vi "VM_ProjetoV4.vi"() -> ()   [LabVIEW 2016]
uses:
  <vilib>/vision/driver/NI_Vision_Acquisition_Software.lvlib
  <resource>/objmgr/imaqdx.rc
  <vilib>/Analysis/NI_AALBase.lvlib
  <vilib>/Analysis/baseanly.llb/Mean (DBL).vi
  <vilib>/userdefined/High Color/IMAQdx.ctl
panel:
  out "Bayer Parameters":T1={"Pattern"=0, "Algorithm"=0, "Red Gain"=1.0, "Green Gain"=1.0, "Blue Gain"=1.0} {"Blue Gain" format="%_4g"; "Green Gain" format="%_4g"; "Red Gain" format="%_4g"; "Algorithm" items=["Bilinear", "VNG"]; "Pattern" items=["GB", "GR", "BG", "RG"]}
  out "output cluster":T2
  in  "Cut Limit":dbl=55.0 format="%#_13g"
  in  "Confirma":bool
  out "Status":string
  out "Câmera Robo":T3(plugin-control)
  out "Câmera Mesa":T3(plugin-control)
  in  "Começa jogada":bool
  in  "stop":bool
  in  "Source Câmera Robo":T4
  in  "Source Câmera Mesa":T4
  out "Dobrao":bool
  out "Passa Vez":bool
  out "place pos Norm":dbl[](array[numeric])
  out "pick pos Norm":dbl[](array[numeric])
  out "place angle":dbl
  out "pick angle":dbl
  # "x 91\ny 176"
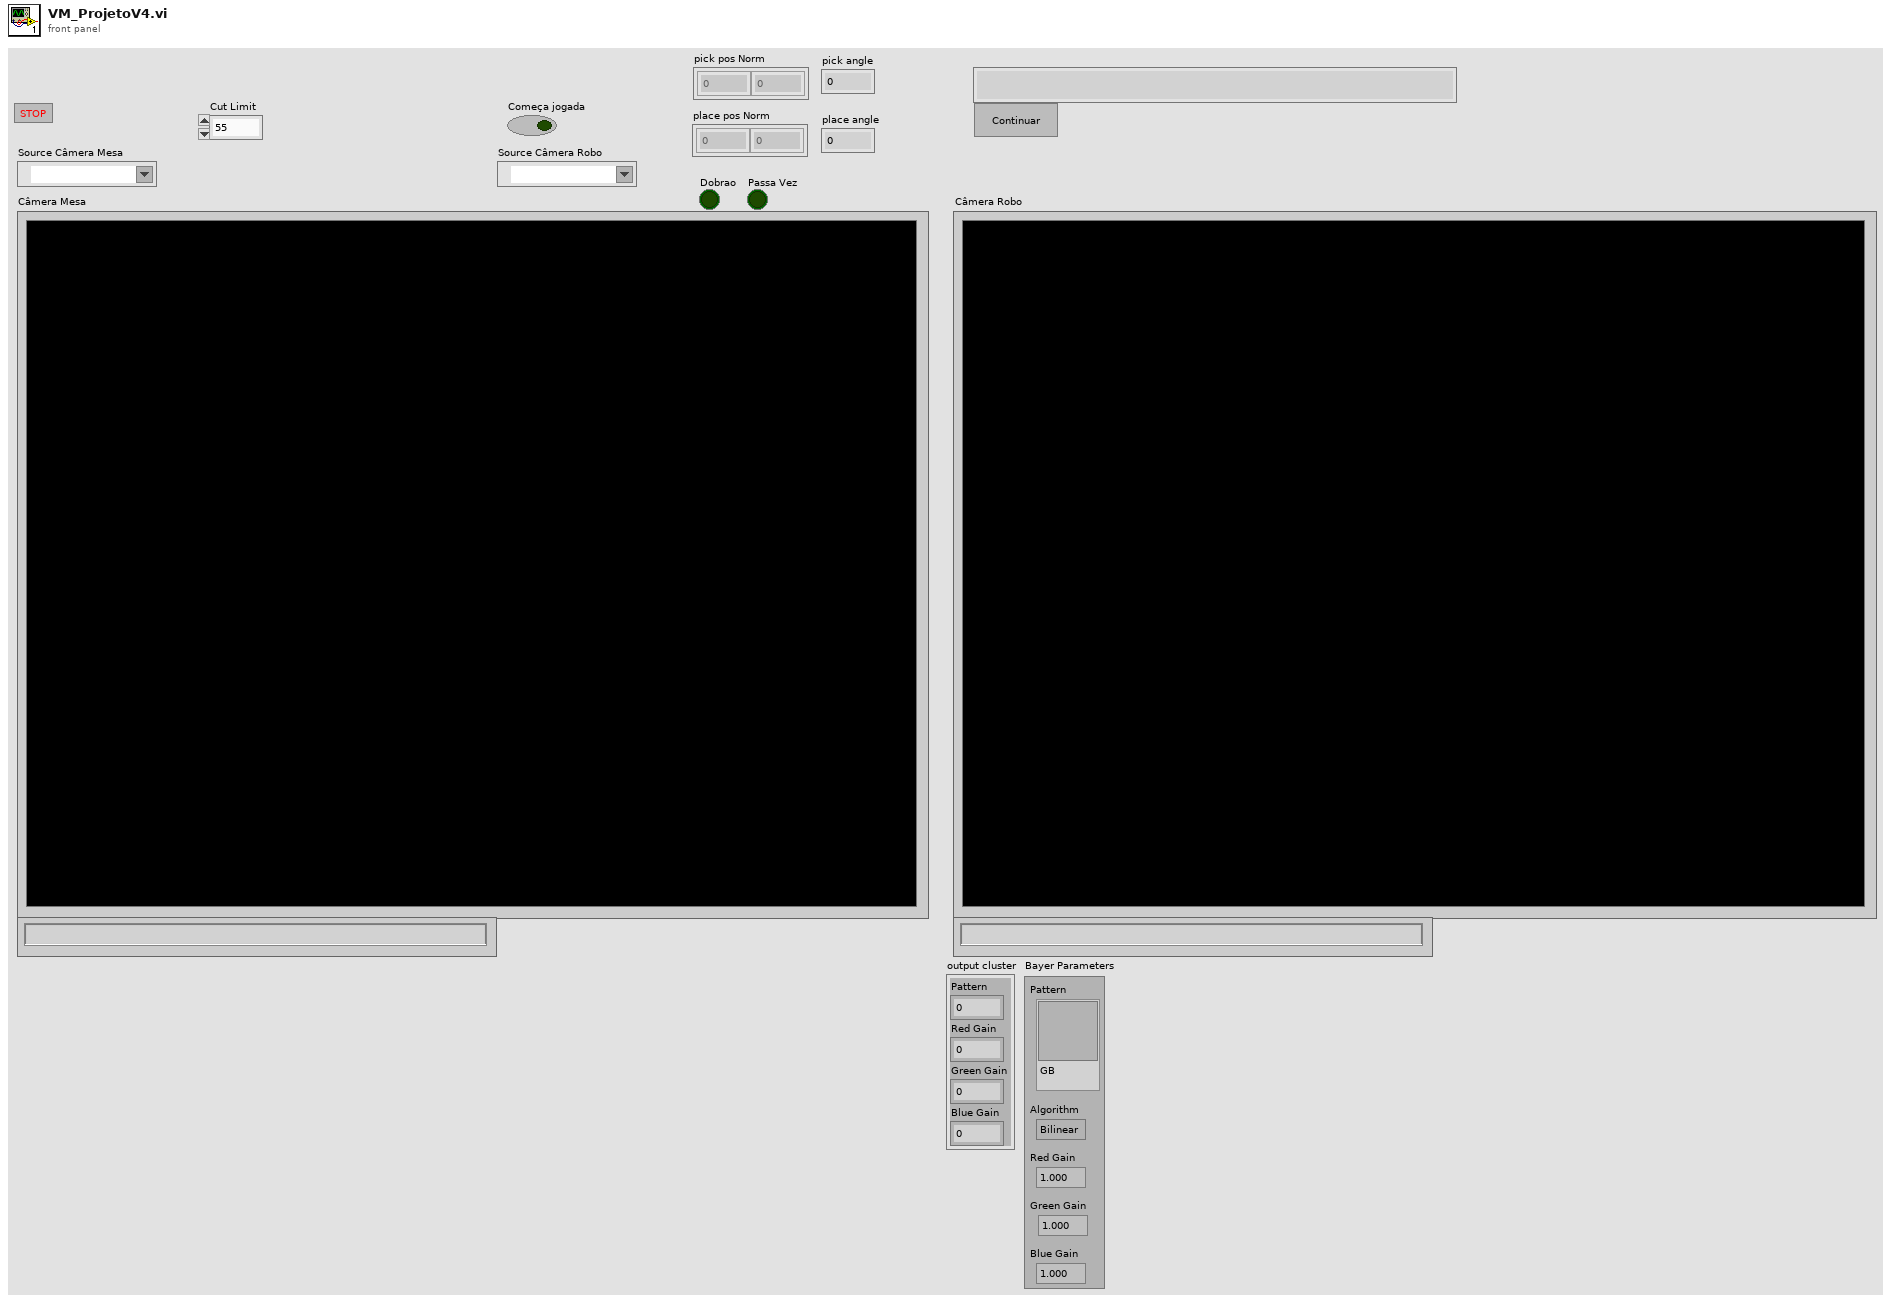
[diagram p1: front panel]
types:
  T1 = cluster{"Pattern":i32, "Algorithm":i32, "Red Gain":dbl, "Green Gain":dbl, "Blue Gain":dbl}
  T2 = cluster{"Pattern":i32, "Red Gain":fxp<+,16,2>, "Green Gain":fxp<+,16,2>, "Blue Gain":fxp<+,16,2>}
  T3 = typedef "IMAQ Image.ctl" = refnum<image>
  T4 = typedef "IMAQdx.ctl" = refnum<k21>
  T5 = typedef "IMAQ Rectangle" = cluster{"Left":i32, "Top":i32, "Right":i32, "Bottom":i32, "Rotation":dbl}
  T6 = typedef "ROI Descriptor" = cluster{"Global Rectangle":i32[], "Contours":cluster{"ID":enum32{"External", "Internal"}, "Type":u32, "Coordinates":i32[]}[]}
  T7 = cluster{"Position":cluster{"x":sgl, "y":sgl}, "Angle":sgl, "Scale":sgl, "Score":sgl, "Bounding Box":cluster{"x":sgl, "y":sgl}[]}[]
  T8 = cluster{"Centro Peça":dbl[], "Centros Númeors":dbl[][], "Números":u8[], "ROI Números":T6[]}[]
  T9 = cluster{"Centro Peça":dbl[], "Centros Númeors":dbl[][], "Números":u8[], "ROI Números":T6[]}
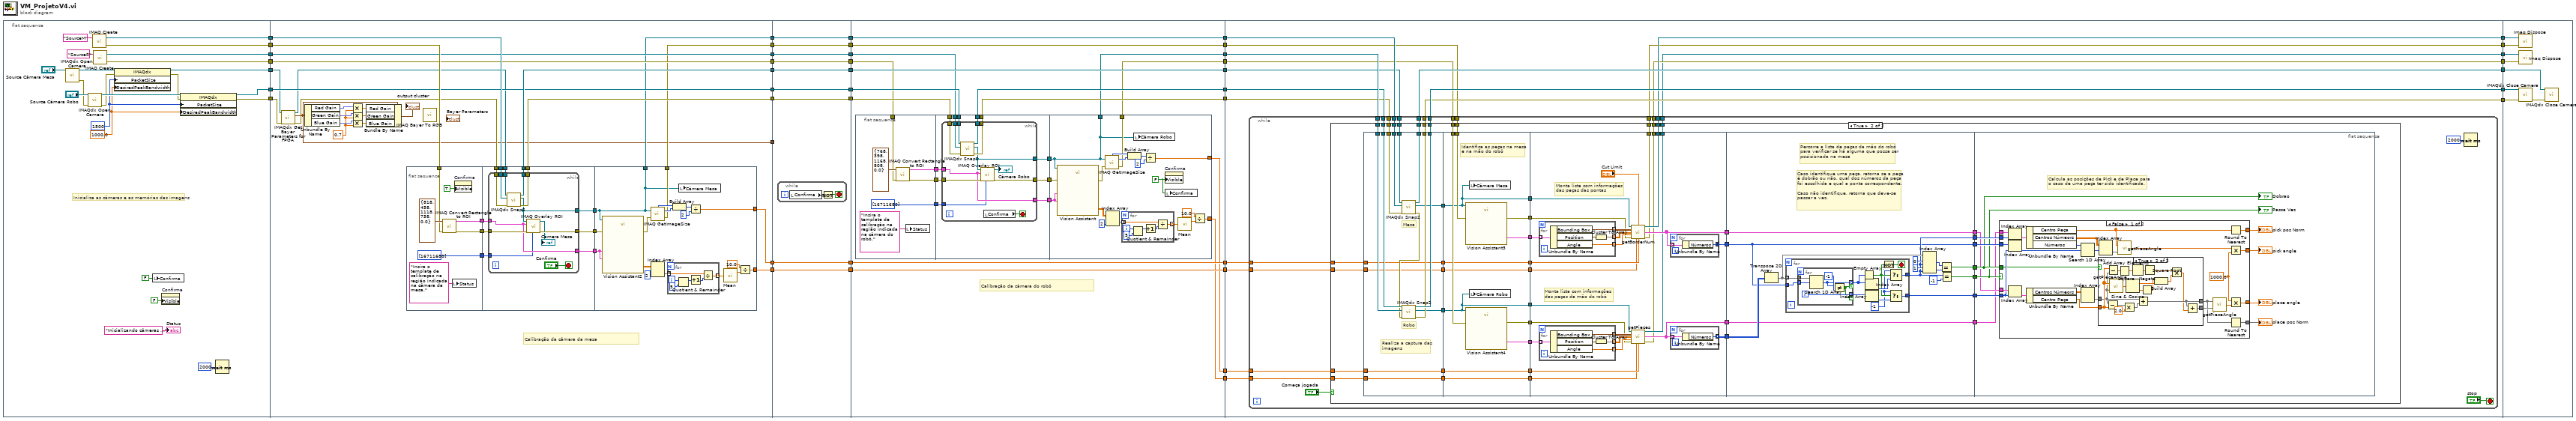
[diagram p0: block diagram]
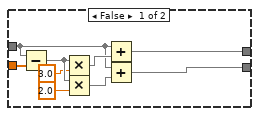
[diagram p3: hidden frame]
diagram:
  n1 = flat-sequence {
    tunnel: [w62] -> w37
    tunnel: [w61] -> w36
    tunnel: [w56] -> w35
    tunnel: [w60] -> w34
    tunnel: [w59] -> w33
    tunnel: [w55] -> w32
    tunnel: [w46] -> w31
    tunnel: w37 -> [w93]
    tunnel: w36 -> [w94]
    tunnel: w35 -> [w79]
    tunnel: w34 -> [w90]
    tunnel: w33 -> [w89]
    tunnel: w32 -> [w77]
    tunnel: [w84] -> w19
    tunnel: [w83] -> w17
    tunnel: [w90] -> w15
    tunnel: [w89] -> w13
    tunnel: [w88] -> w11
    tunnel: [w87] -> w9
    tunnel: w31 -> [w87]
    tunnel: [w86] -> w7
    tunnel: [w81] -> w5
    tunnel: [w80] -> w3
    tunnel: [w68] -> w1
    tunnel: w19 -> [w158]
    tunnel: [w158] -> w18
    tunnel: w17 -> [w157]
    tunnel: [w157] -> w16
    tunnel: w15 -> [w156]
    tunnel: [w156] -> w14
    tunnel: w13 -> [w155]
    tunnel: [w155] -> w12
    tunnel: w11 -> [w154]
    tunnel: [w154] -> w10
    tunnel: w9 -> [w153]
    tunnel: [w153] -> w8
    tunnel: w7 -> [w152]
    tunnel: [w152] -> w6
    tunnel: w5 -> [w151]
    tunnel: [w151] -> w4
    tunnel: w3 -> [w150]
    tunnel: [w150] -> w2
    tunnel: w1 -> [_]
    tunnel: w18 -> [w181]
    tunnel: [w181] -> w30
    tunnel: w16 -> [w180]
    tunnel: [w180] -> w29
    tunnel: w14 -> [w166]
    tunnel: [w165] -> w28
    tunnel: w12 -> [w164]
    tunnel: [w163] -> w27
    tunnel: w10 -> [w179]
    tunnel: [w179] -> w26
    tunnel: w8 -> [w168]
    tunnel: [w167] -> w25
    tunnel: w6 -> [w170]
    tunnel: [w169] -> w24
    tunnel: w4 -> [w178]
    tunnel: [w178] -> w23
    tunnel: w2 -> [w177]
    tunnel: [w177] -> w22
    tunnel: [w162] -> w21
    tunnel: [w161] -> w20
    tunnel: [w249] -> w44
    tunnel: [w252] -> w43
    tunnel: [w246] -> w42
    tunnel: [w251] -> w41
    tunnel: [w250] -> w40
    tunnel: [w248] -> w39
    tunnel: [w247] -> w38
    tunnel: w30 -> [w245]
    tunnel: w29 -> [w244]
    tunnel: w28 -> [w243]
    tunnel: w27 -> [w242]
    tunnel: w26 -> [w241]
    tunnel: w25 -> [w240]
    tunnel: w24 -> [w239]
    tunnel: w23 -> [w237]
    tunnel: w22 -> [w238]
    tunnel: w21 -> [w235]
    tunnel: w20 -> [w236]
    tunnel: w44 -> [w488]
    tunnel: w43 -> [w486]
    tunnel: w42 -> [w490]
    tunnel: w41 -> [w493]
    tunnel: w40 -> [w492]
    tunnel: w39 -> [w489]
    tunnel: w38 -> [w491]
    frame #0 {
      w50 = 1000.0 ("DesiredPeakBandwidth")
      w51 = u32 1500 ("PacketSize")
      # "Inicializa as câmeras e as memórias das imagens"
      n2 = call <vilib>:"IMAQdx Open Camera.vi"("Session In"="Source Câmera Mesa") -> ("error out"=w54:errorcluster, "Session Out"=w57:T4)  [unwired: 9 in]
      n3 = call <vilib>:"IMAQdx Open Camera.vi"("error in"=w54, "Session In"="Source Câmera Robo") -> ("error out"=w53:errorcluster, "Session Out"=w58:T4)  [unwired: 8 in]
      n4 = call "IMAQ Create"("Image Name"="SourceM") -> ("New Image"=w62:T3, "error out"=w61:errorcluster)  [unwired: 4 in]
      n5 = call "IMAQ Create"("Image Name"="SourceR") -> ("New Image"=w60:T3, "error out"=w59:errorcluster)  [unwired: 4 in]
      n6 = property class="IMAQdx"(reference=w57, error in=w53, "PacketSize"=w51, "DesiredPeakBandwidth"=w50) -> (reference out=w56:T4, error out=w52:errorcluster)
      n7 = local write "Confirma"(FALSE ("Confirma")) -> ()
      n8 = property on="Confirma" class="Bool (strict)"("Visible"=FALSE) -> ()  [unwired: 2 in, 2 out]
      n9 = property class="IMAQdx"(reference=w58, error in=w52, "PacketSize"=w51, "DesiredPeakBandwidth"=w50) -> (reference out=w46:T4, error out=w55:errorcluster)
      n10 = Wait (ms)(milliseconds to wait=u32 2000) -> ()  [unwired: 1 out]
      "Status" <- "Inicializando câmeras ..." ("Status")
    }
    frame #1 {
      w69 = 0.7
      # "Calibração da câmera da mesa"
      n11 = call <vilib>:"IMAQdx Get Bayer Parameters for FPGA.vi"("error in (no error)"=w77, "IMAQdx Session In"=w79) -> ("error out"=w76:errorcluster, "Bayer Parameters"=w68:T2, "IMAQdx Session Out"=w78:T4)  [unwired: 7 in]
      n12 = Unbundle By Name(w68) -> ("Red Gain"=w72:fxp<+,16,2>, "Green Gain"=w71:fxp<+,16,2>, "Blue Gain"=w70:fxp<+,16,2>)
      n13 = Multiply(x=w72, y=w69) -> (x*y=w75:dbl)
      n14 = Multiply(x=w71, y=w69) -> (x*y=w74:dbl)
      n15 = Multiply(x=w70, y=w69) -> (x*y=w73:dbl)
      n16 = Bundle By Name(cluster=w68, "Red Gain"=w75, "Green Gain"=w74, "Blue Gain"=w73) -> (→"output cluster":T2)
      n17 = flat-sequence {
        tunnel: w94 -> [w101]
        tunnel: [w99] -> w96
        tunnel: [w98] -> w95
        tunnel: [u32[] [16711680] ("Colors (Green)")] -> w82
        tunnel: w78 -> [w114]
        tunnel: w76 -> [w113]
        tunnel: w93 -> [w112]
        tunnel: [w111] -> w88
        tunnel: [w110] -> w86
        tunnel: w96 -> [w109]
        tunnel: w95 -> [w108]
        tunnel: [w107] -> w92
        tunnel: [w106] -> w91
        tunnel: [w105] -> w85
        tunnel: w82 -> [w104]
        tunnel: w92 -> [w143]
        tunnel: w91 -> [w142]
        tunnel: [w134] -> w81
        tunnel: w85 -> [w127]
        tunnel: [w127] -> w84
        tunnel: [w129] -> w83
        tunnel: [w128] -> w80
        frame #0 {
          n18 = call "IMAQ Convert Rectangle to ROI"("error in (no error)"=w101, "Rectangle"=T5 {"Left"=818, "Top"=458, "Right"=1118, "Bottom"=758, "Rotation"=0.0}) -> ("error out"=w99:errorcluster, "ROI Descriptor"=w98:T6)  [unwired: 7 in]
          n19 = local write "Status"("Insira o template de calibração na região indicada na câmera da mesa." ("Status")) -> ()
          n20 = property on="Confirma" class="Bool (strict)"("Visible"=TRUE) -> ()  [unwired: 2 in, 2 out]
        }
        frame #1 {
          n21 = while {
            tunnel: w114 -> [w125]
            tunnel: w113 -> [w124]
            tunnel: w112 -> [w123]
            tunnel: [w122] -> w111
            tunnel: [w121] -> w110
            tunnel: w109 -> [w120]
            tunnel: w108 -> [w117]
            tunnel: [w119] -> w107
            tunnel: [w117] -> w106
            tunnel: [w116] -> w105
            tunnel: w104 -> [w115]
            stop <- "Confirma" stop-if-true
            n22 = call <vilib>:"IMAQdx Snap2.vi"("error in"=w124, "Image In"=w123, "Session In"=w125) -> ("error out"=w121:errorcluster, "Image Out"=w116:T3, "Session Out"=w122:T4)  [unwired: 6 in]
            n23 = call "IMAQ Overlay ROI"("Colors (Green)"=w115, "error in (no error)"=w120, "ROI Descriptor"=w117, "Image"=w116) -> ("error out"=w119:errorcluster, "Image Out"=→"Câmera Mesa":T3)  [unwired: 6 in]
          }
        }
        frame #2 {
          n24 = call "Vision Assistant2"("Image In"=w127, "ROI Descriptor (Adv. Straight Edge 1)"=w142, "ROI Descriptor (Copy of Adv. Straight Edge 1)"=w142, "error in"=w143) -> ("Caliper Results (Caliper 2)"=w141:sgl[][], "error out"=w135:errorcluster)  [unwired: 21 in, 1 out]
          n25 = call "IMAQ GetImageSize"("Image"=w127, "error in (no error)"=w135) -> ("Y Resolution"=w133:i32, "X Resolution"=w132:i32, "error out"=w129:errorcluster)  [unwired: 2 in]
          n26 = Index Array(array=w141, index (col)=2 ("disabled index (col)")) -> (element=w139:sgl[])  [unwired: 1 in]
          n27 = for {
            tunnel: w139 -> [w146] mode=indexing
            tunnel: [w144] -> w138 mode=indexing
            i -> [w149]
            n28 = Quotient & Remainder(x=w149, y=5) -> (x-y*floor(x/y)=w147:i32)  [unwired: 1 out]
            n29 = Increment(x=w147) -> (x+1=w145:i32)
            n30 = Divide(x=w146, y=w145) -> (x/y=w144:sgl)
          }
          n31 = Build Array(w132, w133) -> (w131:i32[])
          n32 = local write "Câmera Mesa"(w127) -> ()
          n33 = Divide(x=w131, y=2) -> (x/y=w128:dbl[])
          n34 = call-poly <vilib>:"Mean.vi"("X"=w138) -> ("mean"=w137:dbl)  [unwired: 1 out]
          n35 = Divide(x=10.0, y=w137) -> (x/y=w134:dbl)
        }
      }
      n36 = call "IMAQ Bayer To RGB"() -> ()  [unwired: 10 in, 2 out]
    }
    frame #2 {
      n37 = while {
        stop <- w160 stop-if-true
        n38 = local read "Confirma"() -> (w159:bool)
        n39 = Not(x=w159) -> (.not. x?=w160:bool)
      }
    }
    frame #3 {
      # "Calibração da câmera do robô"
      n40 = flat-sequence {
        tunnel: w164 -> [w185]
        tunnel: [w184] -> w176
        tunnel: [w183] -> w175
        tunnel: [u32[] [16711680] ("Colors (Green)")] -> w174
        tunnel: w168 -> [w198]
        tunnel: w170 -> [w197]
        tunnel: w166 -> [w196]
        tunnel: [w195] -> w167
        tunnel: [w194] -> w169
        tunnel: w176 -> [w193]
        tunnel: w175 -> [w192]
        tunnel: [w191] -> w173
        tunnel: [w190] -> w172
        tunnel: [w189] -> w171
        tunnel: w174 -> [w188]
        tunnel: w173 -> [w228]
        tunnel: w172 -> [w227]
        tunnel: [w219] -> w162
        tunnel: w171 -> [w212]
        tunnel: [w212] -> w165
        tunnel: [w214] -> w163
        tunnel: [w213] -> w161
        frame #0 {
          n41 = call "IMAQ Convert Rectangle to ROI"("error in (no error)"=w185, "Rectangle"=T5 {"Left"=768, "Top"=398, "Right"=1168, "Bottom"=808, "Rotation"=0.0}) -> ("error out"=w184:errorcluster, "ROI Descriptor"=w183:T6)  [unwired: 7 in]
          n42 = local write "Status"("Insira o template de calibração na região indicada na câmera do robô." ("Status")) -> ()
        }
        frame #1 {
          n43 = while {
            tunnel: w198 -> [w210]
            tunnel: w197 -> [w209]
            tunnel: w196 -> [w208]
            tunnel: [w207] -> w195
            tunnel: [w206] -> w194
            tunnel: w193 -> [w205]
            tunnel: w192 -> [w203]
            tunnel: [w204] -> w191
            tunnel: [w203] -> w190
            tunnel: [w202] -> w189
            tunnel: w188 -> [w201]
            stop <- w199 stop-if-true
            n44 = call <vilib>:"IMAQdx Snap2.vi"("error in"=w209, "Image In"=w208, "Session In"=w210) -> ("error out"=w206:errorcluster, "Image Out"=w202:T3, "Session Out"=w207:T4)  [unwired: 6 in]
            n45 = call "IMAQ Overlay ROI"("Colors (Green)"=w201, "error in (no error)"=w205, "ROI Descriptor"=w203, "Image"=w202) -> ("error out"=w204:errorcluster, "Image Out"=→"Câmera Robo":T3)  [unwired: 6 in]
            n46 = local read "Confirma"() -> (w199:bool)
          }
        }
        frame #2 {
          w211 = FALSE ("Visible")
          n47 = call "Vision Assistant"("Image In"=w212, "ROI Descriptor (Adv. Straight Edge 1)"=w227, "ROI Descriptor (Copy of Adv. Straight Edge 1)"=w227, "error in"=w228) -> ("Caliper Results (Caliper 2)"=w226:sgl[][], "error out"=w220:errorcluster)  [unwired: 21 in, 1 out]
          n48 = call "IMAQ GetImageSize"("Image"=w212, "error in (no error)"=w220) -> ("Y Resolution"=w218:i32, "X Resolution"=w217:i32, "error out"=w214:errorcluster)  [unwired: 2 in]
          n49 = Index Array(array=w226, index (col)=2 ("disabled index (col)")) -> (element=w224:sgl[])  [unwired: 1 in]
          n50 = for {
            tunnel: w224 -> [w231] mode=indexing
            tunnel: [w229] -> w223 mode=indexing
            i -> [w234]
            n51 = Quotient & Remainder(x=w234, y=5) -> (x-y*floor(x/y)=w232:i32)  [unwired: 1 out]
            n52 = Increment(x=w232) -> (x+1=w230:i32)
            n53 = Divide(x=w231, y=w230) -> (x/y=w229:sgl)
          }
          n54 = Build Array(w217, w218) -> (w216:i32[])
          n55 = local write "Câmera Robo"(w212) -> ()
          n56 = Divide(x=w216, y=2) -> (x/y=w213:dbl[])
          n57 = property on="Confirma" class="Bool (strict)"("Visible"=w211) -> ()  [unwired: 2 in, 2 out]
          n58 = local write "Confirma"(w211) -> ()
          n59 = call-poly <vilib>:"Mean.vi"("X"=w223) -> ("mean"=w222:dbl)  [unwired: 1 out]
          n60 = Divide(x=10.0, y=w222) -> (x/y=w219:dbl)
        }
      }
    }
    frame #4 {
      n61 = while {
        tunnel: w241 -> [w272]
        tunnel: w245 -> [w271]
        tunnel: w243 -> [w270]
        tunnel: w240 -> [w269]
        tunnel: w239 -> [w268]
        tunnel: [w267] -> w252
        tunnel: [w266] -> w251
        tunnel: [w265] -> w250
        tunnel: w244 -> [w264]
        tunnel: w242 -> [w263]
        tunnel: [w262] -> w249
        tunnel: [w261] -> w246
        tunnel: [w259] -> w248
        tunnel: [w258] -> w247
        tunnel: w238 -> [w256]
        tunnel: w237 -> [w255]
        tunnel: w236 -> [w254]
        tunnel: w235 -> [w253]
        stop <- "stop" stop-if-true
        n62 = case shown="True" "Começa jogada" {
          tunnel: w272 -> [w280 w325]
          tunnel: w271 -> [w277 w324]
          tunnel: w270 -> [w276 w323]
          tunnel: w269 -> [w279 w322]
          tunnel: w268 -> [w278 w321]
          tunnel: [w280 w320] -> w267
          tunnel: [w279 w319] -> w266
          tunnel: [w278 w318] -> w265
          tunnel: w264 -> [w275 w316]
          tunnel: w263 -> [w274 w314]
          tunnel: [w277 w303] -> w262
          tunnel: [w276 w302] -> w261
          tunnel: [w275 w294] -> w259
          tunnel: [w274 w293] -> w258
          tunnel: w256 -> [_ w292]
          tunnel: w255 -> [_ w291]
          tunnel: w254 -> [_ w290]
          tunnel: w253 -> [_ w289]
          frame False {
          }
          frame True {
            n63 = flat-sequence {
              tunnel: w325 -> [w340]
              tunnel: w324 -> [w339]
              tunnel: w323 -> [w338]
              tunnel: w322 -> [w337]
              tunnel: w321 -> [w331]
              tunnel: [w336] -> w320
              tunnel: [w335] -> w319
              tunnel: [w334] -> w318
              tunnel: [w333] -> w317
              tunnel: [w332] -> w315
              tunnel: w292 -> [w329]
              tunnel: w291 -> [w328]
              tunnel: w290 -> [w327]
              tunnel: w289 -> [w326]
              tunnel: [w329] -> w287
              tunnel: [w328] -> w285
              tunnel: [w327] -> w283
              tunnel: [w326] -> w282
              tunnel: w317 -> [w342]
              tunnel: w316 -> [w352]
              tunnel: w315 -> [w341]
              tunnel: w314 -> [w351]
              tunnel: [w350] -> w313
              tunnel: [w349] -> w312
              tunnel: [w341] -> w311
              tunnel: [w342] -> w310
              tunnel: [w348] -> w309
              tunnel: [w347] -> w308
              tunnel: [w346] -> w288
              tunnel: w287 -> [w346]
              tunnel: [w345] -> w286
              tunnel: w285 -> [w345]
              tunnel: [w344] -> w284
              tunnel: w283 -> [w344]
              tunnel: w282 -> [w343]
              tunnel: [w343] -> w281
              tunnel: w313 -> [w377]
              tunnel: w312 -> [w376]
              tunnel: w311 -> [w366]
              tunnel: w310 -> [w371]
              tunnel: w309 -> [w372]
              tunnel: w308 -> [w367]
              tunnel: [w365] -> w307
              tunnel: [w364] -> w306
              tunnel: [w363] -> w305
              tunnel: [w362] -> w304
              tunnel: [w361] -> w303
              tunnel: [w360] -> w302
              tunnel: [w359] -> w294
              tunnel: [w358] -> w293
              tunnel: w288 -> [w357]
              tunnel: w286 -> [w356]
              tunnel: w284 -> [w355]
              tunnel: w281 -> [w354]
              tunnel: w307 -> [w392]
              tunnel: w306 -> [w399]
              tunnel: w305 -> [w398]
              tunnel: w304 -> [w394]
              tunnel: [w398] -> w301
              tunnel: [w397] -> w300
              tunnel: [w396] -> w299
              tunnel: [w395] -> w298
              tunnel: [w394] -> w297
              tunnel: [w393] -> w296
              tunnel: [w392] -> w295
              tunnel: w301 -> [w425]
              tunnel: w300 -> [w427]
              tunnel: w299 -> [w426]
              tunnel: w298 -> [w433]
              tunnel: w297 -> [w424]
              tunnel: w296 -> [w432]
              tunnel: w295 -> [w431]
              frame #0 {
                # "Realiza a captura das\nimagens"
                # "Robo"
                # "Mesa"
                n64 = call <vilib>:"IMAQdx Snap2.vi"("error in"=w331, "Image In"=w339, "Session In"=w340) -> ("error out"=w330:errorcluster, "Image Out"=w333:T3, "Session Out"=w336:T4)  [unwired: 6 in]
                n65 = call <vilib>:"IMAQdx Snap2.vi"("error in"=w330, "Image In"=w338, "Session In"=w337) -> ("error out"=w334:errorcluster, "Image Out"=w332:T3, "Session Out"=w335:T4)  [unwired: 6 in]
              }
              frame #1 {
                # "Identifica as peças na mesa\ne na mão do robô"
                n66 = call "Vision Assistant3"("Image In"=w342, "error in"=w352) -> ("Matches (Pattern Matching 1)"=w349:T7, "error out"=w348:errorcluster)  [unwired: 23 in, 1 out]
                n67 = call "Vision Assistant4"("Image In"=w341, "error in"=w351) -> ("Matches (Pattern Matching 1)"=w350:T7, "error out"=w347:errorcluster)  [unwired: 23 in, 1 out]
                n68 = local write "Câmera Mesa"(w342) -> ()
                n69 = local write "Câmera Robo"(w341) -> ()
              }
              frame #2 {
                # "Monta lista com informações\ndas peças das pontas"
                # "Monta lista com informações\ndas peças da mão do robô"
                n70 = for {
                  tunnel: w376 -> [w386] mode=indexing
                  tunnel: [w384] -> w374 mode=indexing
                  tunnel: [w383] -> w375 mode=indexing
                  tunnel: [w382] -> w373 mode=indexing
                  n71 = Unbundle By Name(w386) -> ("Bounding Box"=w383:cluster{"x":sgl, "y":sgl}[], "Position"=w385:cluster{"x":sgl, "y":sgl}, "Angle"=w382:sgl)
                  n72 = Cluster To Array(cluster=w385) -> (array=w384:sgl[])
                }
                n73 = for {
                  tunnel: w377 -> [w391] mode=indexing
                  tunnel: [w389] -> w369 mode=indexing
                  tunnel: [w388] -> w370 mode=indexing
                  tunnel: [w387] -> w368 mode=indexing
                  n74 = Unbundle By Name(w391) -> ("Bounding Box"=w388:cluster{"x":sgl, "y":sgl}[], "Position"=w390:cluster{"x":sgl, "y":sgl}, "Angle"=w387:sgl)
                  n75 = Cluster To Array(cluster=w390) -> (array=w389:sgl[])
                }
                n76 = call "getBorderNum.vi"("Refnum in"=w371, "Cut Limit"="Cut Limit", "Bounding Box"=w375, "Position"=w374, "Angle"=w373, "error in (no error)"=w372, "Step"=w356, "Origin Pixel"=w357) -> ("Refnum out"=w361:T3, "Data Pieces"=w363:T8, "error out"=w359:errorcluster)  [unwired: 5 in]
                n77 = call "getPieces.vi"("Refnum in"=w366, "Bounding Box"=w370, "Position"=w369, "Angle"=w368, "error in (no error)"=w367, "Step"=w354, "Origin Pixel"=w355) -> ("Refnum out"=w360:T3, "Data Pieces"=w362:T8, "error out"=w358:errorcluster)  [unwired: 6 in]
                n78 = for {
                  tunnel: w363 -> [w381] mode=indexing
                  tunnel: [w380] -> w365 mode=concatenating
                  n79 = Unbundle By Name(w381) -> ("Números"=w380:u8[])
                }
                n80 = for {
                  tunnel: w362 -> [w379] mode=indexing
                  tunnel: [w378] -> w364 mode=indexing
                  n81 = Unbundle By Name(w379) -> ("Números"=w378:u8[])
                }
              }
              frame #3 {
                # "Caso identifique uma peça, retorna se a peça\né dobrão ou não, qual dos números da peça\nfoi escolhida e qual a ponta correspondente.\n\nCaso não identifique, retorna que deve-se\npassar a vez."
                # "Percorre a lista de peças da mão do robô\npara verificar se há alguma que possa ser\nposicionada na mesa"
                n82 = Transpose 2D Array(2D array=w399) -> (transposed array=w401:u8[][])
                n83 = for {
                  tunnel: w401 -> [w416] mode=indexing
                  tunnel: w392 -> [w415]
                  tunnel: [w407] -> w395
                  tunnel: [w406] -> w393
                  stop <- w411 stop-if-true
                  w408 = -1 ("t")
                  n84 = for {
                    tunnel: w416 -> [w422]
                    tunnel: w415 -> [w421] mode=indexing
                    tunnel: [w419] -> w413 mode=indexing if=w417
                    tunnel: [w418] -> w412 mode=indexing if=w417
                    i -> [w418]
                    n85 = Search 1D Array(1D array=w422, element=w421) -> (index of element=w419:i32)  [unwired: 1 in]
                    n86 = Not Equal?(x=w419, y=-1) -> (x != y?=w417:bool)
                  }
                  n87 = Empty Array?(array=w413) -> (empty?=w409:bool)
                  n88 = Index Array(array=w413) -> (element=w414:i32)  [unwired: 1 in]
                  n89 = Index Array(array=w412) -> (element=w410:i32)  [unwired: 1 in]
                  n90 = Not(x=w409) -> (.not. x?=w411:bool)
                  n91 = Select(t=w408, s=w409, f=w414) -> (s? t:f=w406:i32)
                  n92 = Select(t=w408, s=w409, f=w410) -> (s? t:f=w407:i32)
                }
                n93 = Index Array(array=w401, index (row) #1=0 ("disabled index (row)"), index (col) #1=w393, index (row) #2=1 ("disabled index (row)"), index (col) #2=w393) -> (element #1=w405:u8, element #2=w404:u8)
                n94 = Equal?(x=w405, y=w404) -> (x = y?=w397:bool)
                n95 = Equal?(x=w393, y=-1) -> (x = y?=w396:bool)
              }
              frame #4 {
                # "Calcula as posições de Pick e de Place para\no caso de uma peça ter sido identificada."
                n96 = case shown="False" w426 {
                  tunnel: w424 -> [w455 _]
                  tunnel: w432 -> [w454 _]
                  tunnel: w433 -> [w451 _]
                  tunnel: w425 -> [w453 _]
                  tunnel: w431 -> [w443 _]
                  tunnel: w427 -> [w448 _]
                  tunnel: [w437 _] -> w423
                  tunnel: [w436 _] -> w430
                  tunnel: [w439 _] -> w429
                  tunnel: [w441 _] -> w428
                  frame False {
                    w438 = 1000.0
                    n97 = Index Array(array=w455, index=w454) -> (element=w456:T9)
                    n98 = Index Array(array=w443, index=w451) -> (element=w450:u8)
                    n99 = Index Array(array=w453, index=w451) -> (element=w452:T9)
                    n100 = Unbundle By Name(w456) -> ("Centro Peça"=w434:dbl[], "Centros Númeors"=w458:dbl[][], "Números"=w457:u8[])
                    n101 = Unbundle By Name(w452) -> ("Centros Númeors"=w445:dbl[][], "Centro Peça"=w444:dbl[])
                    n102 = Search 1D Array(1D array=w457, element=w450) -> (index of element=w459:i32)  [unwired: 1 in]
                    n103 = Index Array(array=w445) -> (element=w447:dbl[])  [unwired: 2 in]
                    n104 = case shown="True" w448 {
                      tunnel: w447 -> [w463 w478]
                      tunnel: w444 -> [w467 w479]
                      tunnel: [w461 w471] -> w446
                      tunnel: [w460 w470] -> w435
                      frame False {
                        n105 = Subtract(x=w463, y=w467) -> (x-y=w466:dbl[])
                        n106 = Multiply(x=w466, y=3.0) -> (x*y=w468:dbl[])
                        n107 = Multiply(x=w466, y=2.0) -> (x*y=w462:dbl[])
                        n108 = Add(x=w463, y=w468) -> (x+y=w460:dbl[])
                        n109 = Add(x=w463, y=w462) -> (x+y=w461:dbl[])
                      }
                      frame True {
                        n110 = Subtract(x=w478, y=w479) -> (x-y=w485:dbl[])
                        n111 = Subtract(x=w479, y=w478) -> (x-y=w482:dbl[])
                        n112 = call "getPieceAngle.vi"("Center Num"=w478, "Center Piece"=w479) -> ("Angle"=w477:dbl)
                        n113 = Square(x=w482) -> (x^2=w481:dbl[])
                        n114 = Multiply(x=w485, y=2.0) -> (x*y=w483:dbl[])
                        n115 = Sine & Cosine(0:w477) -> (1:w475:dbl, 2:w476:dbl)
                        n116 = Add Array Elements(numeric array=w481) -> (sum=w480:dbl)
                        n117 = Add(x=w478, y=w483) -> (x+y=w470:dbl[])
                        n118 = Negate(x=w476) -> (-x=w474:dbl)
                        n119 = Square Root(x=w480) -> (sqrt(x)=w472:dbl)
                        n120 = Build Array(w474, w475) -> (w473:dbl[])
                        n121 = Multiply(x=w472, y=w473) -> (x*y=w469:dbl[])
                        n122 = Add(x=w470, y=w469) -> (x+y=w471:dbl[])
                      }
                    }
                    n123 = Index Array(array=w458, index (row)=w459) -> (element=w449:dbl[])  [unwired: 1 in]
                    n124 = call "getPieceAngle.vi"("Center Num"=w449, "Center Piece"=w434) -> ("Angle"=w442:dbl)
                    n125 = call "getPieceAngle.vi"("Center Num"=w446, "Center Piece"=w435) -> ("Angle"=w440:dbl)
                    n126 = Round To Nearest(number=w434) -> (nearest integer value=w437:dbl[])
                    n127 = Multiply(x=w442, y=w438) -> (x*y=w441:dbl)
                    n128 = Multiply(x=w438, y=w440) -> (x*y=w439:dbl)
                    n129 = Round To Nearest(number=w435) -> (nearest integer value=w436:dbl[])
                  }
                  frame True {
                  }
                }
                "pick angle" <- w428
                "pick pos Norm" <- w423
                "place angle" <- w429
                "place pos Norm" <- w430
                "Passa Vez" <- w426
                "Dobrao" <- w427
              }
            }
          }
        }
        n130 = Wait (ms)(milliseconds to wait=u32 2000) -> ()  [unwired: 1 out]
      }
    }
    frame #5 {
      n131 = call "Imaq Dispose"("Image"=w488, "error in (no error)"=w489) -> ()  [unwired: 4 in, 1 out]
      n132 = call "Imaq Dispose"("Image"=w490, "error in (no error)"=w491) -> ()  [unwired: 4 in, 1 out]
      n133 = call <vilib>:"IMAQdx Close Camera.vi"("error in"=w492, "Session In"=w493) -> ("error out"=w487:errorcluster)  [unwired: 9 in]
      n134 = call <vilib>:"IMAQdx Close Camera.vi"("error in"=w487, "Session In"=w486) -> ()  [unwired: 9 in, 1 out]
    }
  }
